vi "ArmCalculateSpeakerShootAngle.vi"() -> (3 "ArmAngle (degrees)":dbl)   [LabVIEW 2023]
doc: "Gets angle to shoot into speaker based on distance from speaker using equation derived from testing\n\nInputs:\n--NONE\nOutputs:\n--ArmAngle--degrees--numeric"
uses:
  <vilib>/Rock Robotics/WPI/ThirdParty/JAS_Junk/TrajLib/TypeDef/X_Y_PAIR.ctl
  <vilib>/Rock Robotics/WPI/ThirdParty/JAS_Junk/TrajLib/VI/FunctionGenerator_New.vi
  <vilib>/Rock Robotics/WPI/ThirdParty/JAS_Junk/TrajLib/VI/FunctionGenerator_Calculate.vi
  <vilib>/gmath/interp.llb/Search Ordered Table.vi
  <vilib>/Rock Robotics/WPI/ThirdParty/JAS_Junk/TrajLib/Trajectory_Library.lvlib
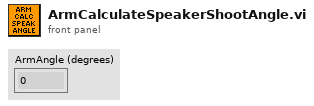
[diagram p1: front panel]
types:
  T1 = typedef "Trajectory_Library.lvlib/X_Y_PAIR.ctl" = cluster{"X":dbl, "Y":dbl}
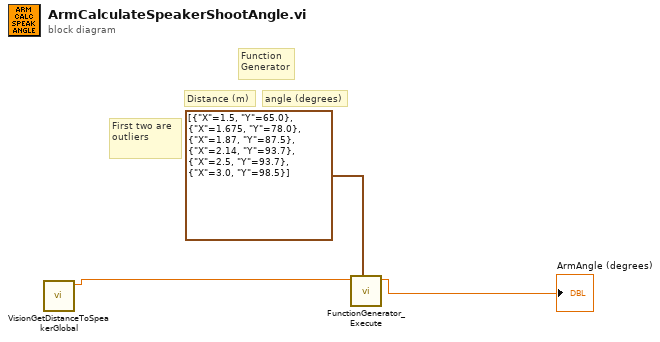
[diagram p0: block diagram]
diagram:
  # "First two are outliers"
  # "Function\nGenerator"
  # "angle (degrees)"
  # "Distance (m)"
  n1 = call "VisionGetDistanceToSpeakerGlobal.vi"() -> ("DistanceFromSpeaker(m)"=w2:dbl)  [unwired: 11 in]
  n2 = call <vilib>:"FunctionGenerator_Execute.vi"("X Y Pairs"=T1[] [{"X"=1.5, "Y"=65.0}, {"X"=1.675, "Y"=78.0}, {"X"=1.87, "Y"=87.5}, {"X"=2.14, "Y"=93.7}, {"X"=2.5, "Y"=93.7}, {"X"=3.0, "Y"=98.5}], "Input Value"=w2) -> ("Output Value"=→"ArmAngle (degrees)":dbl)  [unwired: 9 in]
